vi "Elevator - State Entry.vi"(8 "error in (no error)":errorcluster, 11 "View Model":T1) -> (0 "error out":errorcluster, 3 "View Model":T1)   [LabVIEW 2017]
doc: "Perform actions before calling specific state"
uses:
  View Model/Controls/View Model.ctl
  Configuration/Controls/Config Model.ctl
  Configuration/Controls/Config Data.ctl
  Error Handler/Controls/Error Model.ctl
  Error Handler/Controls/Error Data.ctl
  Error Handler/Controls/Error Type.ctl
  View Model/Controls/Shared Model.ctl
  Controls/Elevator Model.ctl
  Controls/Elevator Location.ctl
  Controls/Elevator CMD Data.ctl
  Controls/Elevator Commands.ctl
  Controls/Elevator Overhead.ctl
  Controls/Elevator States.ctl
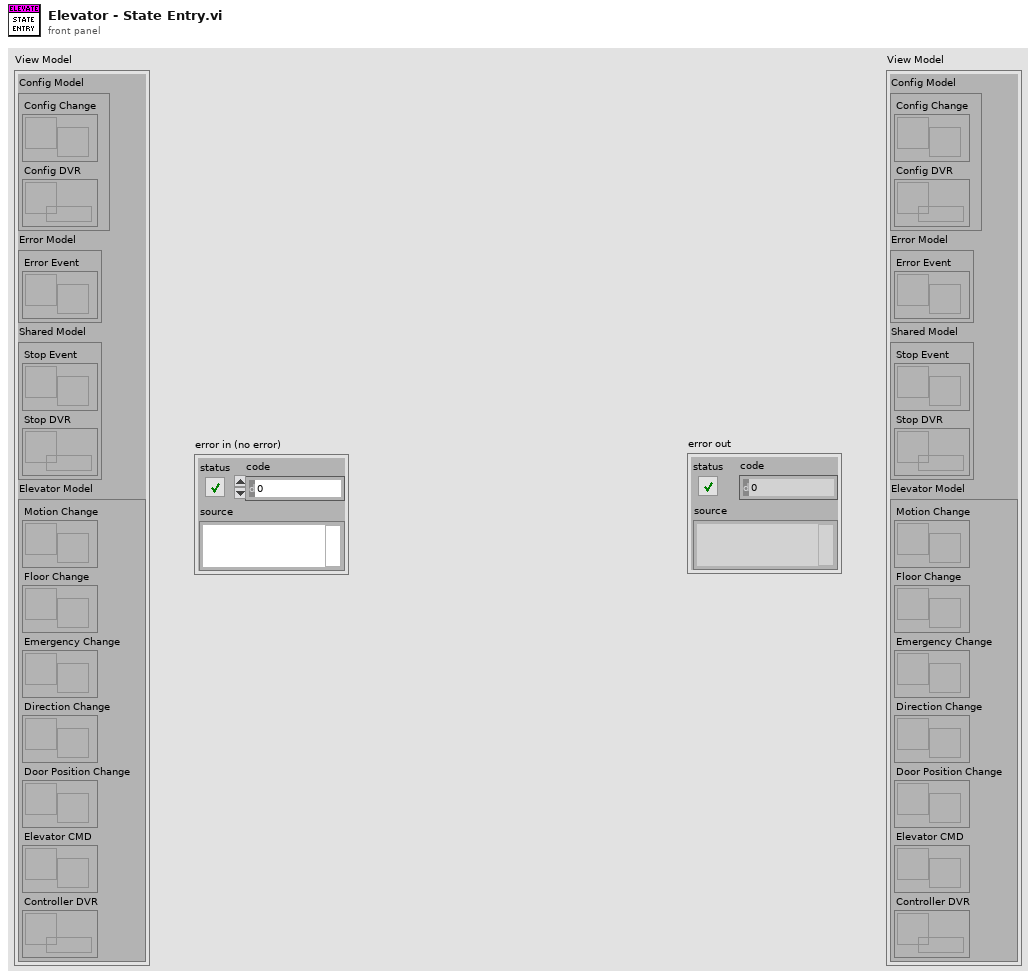
[diagram p1: front panel]
types:
  T1 = typedef "View Model.ctl" = cluster{"Config Model":T2, "Error Model":T3, "Shared Model":T4, "Elevator Model":T5}
  T2 = typedef "Config Model.ctl" = cluster{"Config Change":refnum<user-event>, "Config DVR":refnum<data-value>}
  T3 = typedef "Error Model.ctl" = cluster{"Error Event":refnum<user-event>}
  T4 = typedef "Shared Model.ctl" = cluster{"Stop Event":refnum<user-event>, "Stop DVR":refnum<data-value>}
  T5 = typedef "Elevator Model.ctl" = cluster{"Motion Change":refnum<user-event>, "Floor Change":refnum<user-event>, "Emergency Change":refnum<user-event>, "Direction Change":refnum<user-event>, "Door Position Change":refnum<user-event>, "Elevator CMD":refnum<user-event>, "Controller DVR":refnum<data-value>}
  T6 = typedef "Elevator States.ctl" = enum16{"Initial", "Wait for 1st Request", "Start and Move", "Analysis", "Continue Travel", "Stop at Floor", "Open and Close Door", "No Request", "Emergency", "Terminate"}
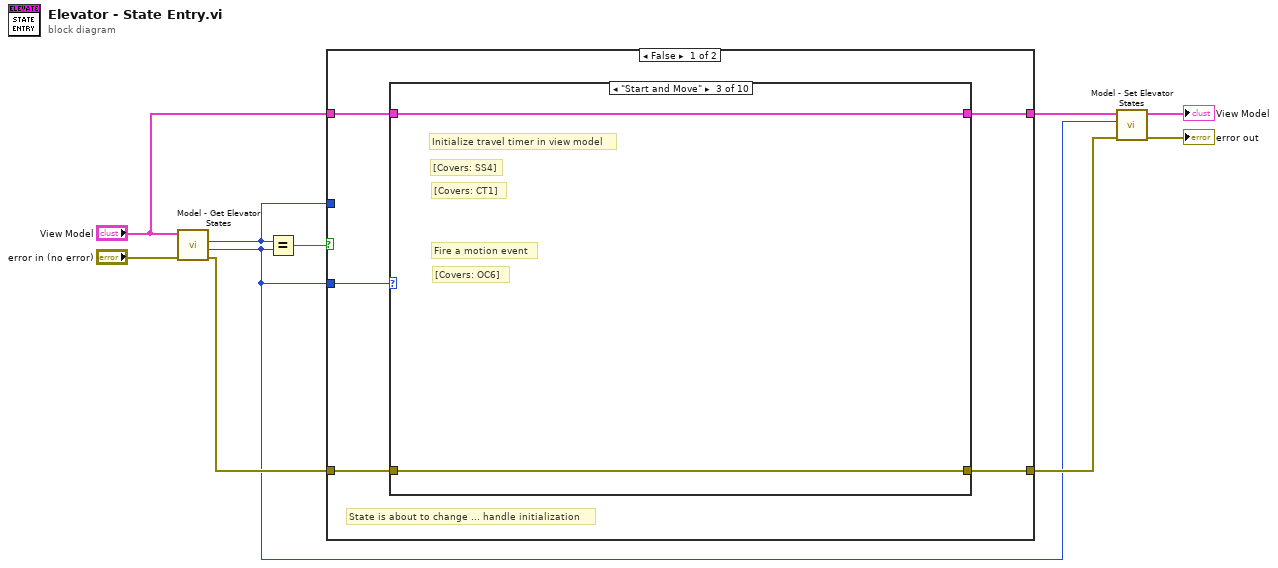
[diagram p0: block diagram]
diagram:
  n1 = call "Model - Get Elevator States.vi"("error in (no error)"="error in (no error)", "View Model"="View Model") -> ("error out"=w6:errorcluster, "Elevator Next State"=w1:T6, "Elevator State"=w9:T6)  [unwired: 6 in, 1 out]
  n2 = Equal?(x=w9, y=w1) -> (x = y?=w10:bool)
  n3 = case shown="False" w10 {
    tunnel: w9 -> [_ _]
    tunnel: w1 -> [w15 _]
    tunnel: "View Model" -> [w14 w37]
    tunnel: [w13 w37] -> w5
    tunnel: w6 -> [w12 w36]
    tunnel: [w11 w36] -> w4
    frame False {
      # "State is about to change ... handle initialization"
      n4 = case shown="\"Start and Move\"" w15 {
        tunnel: w14 -> [w17 w19 w21 w23 w25 w27 w29 w31 w33 w35]
        tunnel: [w17 w19 w21 w23 w25 w27 w29 w31 w33 w35] -> w13
        tunnel: w12 -> [w16 w18 w20 w22 w24 w26 w28 w30 w32 w34]
        tunnel: [w16 w18 w20 w22 w24 w26 w28 w30 w32 w34] -> w11
        frame "Initial", Default {
          # "[Covers: WS1]"
          # "#TODO\nMaintain initial state until Elevator call"
        }
        frame "Wait for 1st Request" {
        }
        frame "Start and Move" {
          # "[Covers: OC6]"
          # "Fire a motion event"
          # "[Covers: CT1]"
          # "[Covers: SS4]"
          # "Initialize travel timer in view model"
        }
        frame "Analysis" {
        }
        frame "Continue Travel" {
        }
        frame "Stop at Floor" {
        }
        frame "Open and Close Door" {
          # "[Covers: OC3A]"
          # "[Covers: OC3]"
          # "Start open door timer"
        }
        frame "No Request" {
        }
        frame "Emergency" {
        }
        frame "Terminate" {
        }
      }
    }
    frame True {
    }
  }
  n5 = call "Model - Set Elevator States.vi"("error in (no error)"=w4, "Elevator State"=w1, "View Model"=w5) -> ("error out"=→"error out":errorcluster, "View Model"=→"View Model":T1)  [unwired: 7 in]
